vi "Read Series.vi"(8 "error in (no error)":errorcluster, 11 "Astromech droid in":refnum<class "Astromech droid.lvclass">) -> (0 "error out":errorcluster, 2 "Series":T1(ring), 3 "Astromech droid out":refnum<class "Astromech droid.lvclass">)   [LabVIEW 2021, in "Astromech droid.lvclass"]
uses:
  Astromech droid.lvclass
  Astromech droid.lvclass/Astromech droid.ctl
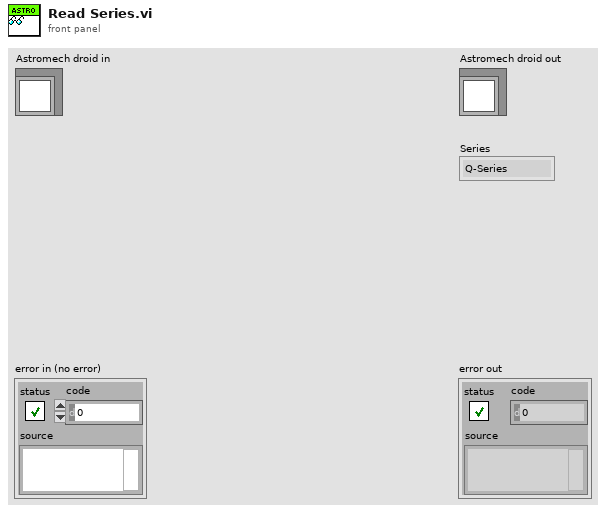
[diagram p1: front panel]
types:
  T1 = enum16{"Q-Series", "BB-Series", "C-Series", "R-Series"}
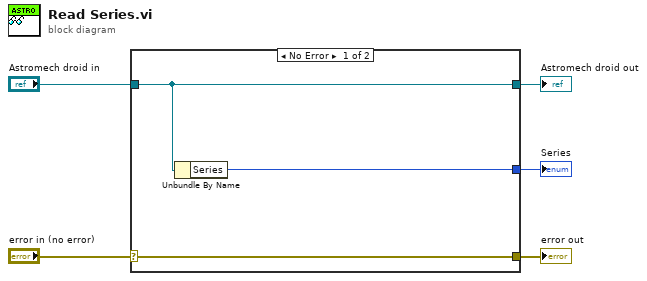
[diagram p0: block diagram]
diagram:
  n1 = case shown="No Error" "error in (no error)" {
    selector: "error in (no error)" -> [w8 w9]
    tunnel: [w8 w9] -> w4
    tunnel: [w7 w10] -> w2
    tunnel: "Astromech droid in" -> [w7 w10]
    tunnel: [w6 _] -> w1
    frame No Error {
      n2 = Unbundle By Name(w7) -> ("Series"=w6:T1)
    }
    frame Error {
    }
  }
  "error out" <- w4
  "Astromech droid out" <- w2
  "Series" <- w1
